vi "FGV PMA Kalibrieren.vi"(8 "GT?":bool, 10 "Aktionen PMA kalibrieren":T1, 11 "Sprachliste":string[][](array[string])) -> (1 "Zustand PMA":string, 2 "Aktionen PMA kalibrieren":T1)   [LabVIEW 2020, in "Auto Kalibrieren.lvlib"]
uses:
  Auto Kalibrieren.lvlib
  Aktionen PMA kalibrieren.ctl
  Aktion FGV CalZustand.ctl
  Analysator Definition/FGV Analysator Definition Aktionen.ctl
  Seiten/CalGas Aufschaltung/FGV CalGas Aktionen.ctl
  Seiten/EL3000/PMA/Aktion FGV Messwerte.ctl
  Aktionen FGV Zustand Kalibrierung.ctl
  Aktionen FGV AutoKAL Daten.ctl
  Seiten/EL3000/Allgemeine VI/FGV Uras26 Aktion.ctl
  Seiten/EL3000/PMA/Kalibrieren/Kalibrierung O2.ctl
  Seiten/EL3000/PMA/PMA.lvlib
  Seiten/EL3000/PMA/Kalibrieren/Kalibrieren.lvlib
  Seiten/EL3000/Allgemeine VI/Allgemeine VI.lvlib
  Analysator Definition/Analysator Definition.lvlib
  Seiten/CalGas Aufschaltung/CalGas Aufschaltung.lvlib
  Linearisierung V2/Linearisierung v2.lvlib
  Sprachverwaltung/Sprachverwaltung.lvlib
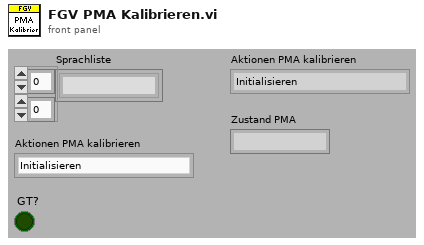
[diagram p1: front panel]
types:
  T1 = typedef "Auto Kalibrieren.lvlib/Aktionen PMA kalibrieren.ctl" = enum16{"Initialisieren", "Warten auf FT-IR", "Anstehende Störung", "0-Gas Aufschalten", "Nullpunkt Anfordern", "Nullpunkt", "Warten auf andere Messgeräte", "Messgas Aufschalten", "Endpunkt Anfordern", "Endpunkt", "Fertig", "Speichern"}
  T2 = typedef "Auto Kalibrieren.lvlib/Aktion FGV CalZustand.ctl" = enum16{"lesen", "Cal FTIR", "Cal FID CH4", "Cal PMA", "init", "Cal FID THC", "THC CG Eingang"}
  T3 = typedef "Analysator Definition.lvlib/FGV Analysator Definition Aktionen.ctl" = enum16{"lesen", "MB setzen", "MB KAL setzen", "laden"}
  T4 = typedef "CalGas Aufschaltung.lvlib/FGV CalGas Aktionen.ctl" = enum16{"lesen", "Analysator Auswahl", "Def.CalGas", "Aufschaltung CalGas", "laden", "speichern", "KAL extrahieren"}
  T5 = typedef "ABB-EL3000.lvlib/PMA.lvlib/Aktion FGV Messwerte.ctl" = enum16{"lesen", "Messwerte", "Messbereich", "Status", "Diagnose Werte"}
  T6 = typedef "Auto Kalibrieren.lvlib/Aktionen FGV Zustand Kalibrierung.ctl" = enum16{"lesen", "LÖSCHEN", "Hintergrund fertig", "Nullpunkt NDIR CO lo", "Endpunkt NDIR CO lo", "Nullpunkt NDIR CO hi", "Endpunkt NDIR CO hi", "Nullpunkt NDIR CO2 lo", "Endpunkt NDIR CO2 lo", "Nullpunkt FID CH4", "Endpunkt FID CH4", "Nullpunkt FID THC", "Endpunkt FID THC", "Nullpunkt PMA", "Endpunkt PMA", "Fehler FT-IR", "Fehler NDIR lo", "Fehler FID CH4", "Fehler FID THC", "Fehler PMA", "TIMEOUT"}
  T7 = typedef "Auto Kalibrieren.lvlib/Aktionen FGV AutoKAL Daten.ctl" = enum16{"lesen", "laden", "speichern", "Aufschaltzeit"}
  T8 = typedef "ABB-EL3000.lvlib/PMA.lvlib/Kalibrieren.lvlib/Kalibrierung O2.ctl" = enum16{"Nullpunkt O2", "Endpunkt O2"}
  T9 = typedef "ABB-EL3000.lvlib/Allgemeine VI.lvlib/FGV Uras26 Aktion.ctl" = enum16{"lesen", "CAL-Daten laden", "Messen", "Kalibrieren vorbereiten", "Kalibrieren", "CAL-Daten speichern", "Toleranz schreiben", "CAL-Daten kopieren"}
  T10 = typedef "Analysator Definition.lvlib/Betriebsdaten Komponente.ctl" = cluster{"Namen":string[], "MB Namen":string[], "Einheit":string, "MB Aktuell":u16, "MB Endwert":u16, "CalGase":u16[], "MB für KAL":u16[], "CG für KAL":u16[]}
  T11 = typedef "CalGas Aufschaltung.lvlib/Aufschaltung CalGas.ctl" = cluster{"Kalibriergas":T12, "Aufschaltpunkt":T13, "Analysator":T14}
  T12 = typedef "Auswahlfeld.ctl" = u16
  T13 = typedef "CalGas Aufschaltung.lvlib/Auswahl Aufschaltpunkt.ctl" = enum16{"über Filterblock", "Analysator direkt", "über PNS", "Entnahme", "Gasdivider"}
  T14 = typedef "CalGas Aufschaltung.lvlib/Auswahl Analysator.ctl" = enum16{"FT-IR", "FID", "PMA", "PMA/FID/FT-IR"}
  T15 = cluster{"Ausfall":bool, "Funktionskontrolle":bool, "Wartungsbedarf":bool}
  T16 = typedef "Auto Kalibrieren.lvlib/Auschaltzeiten Null Endpunktgase.ctl" = cluster{"CO lo 0":sgl, "CO lo E":sgl, "CO hi 0":sgl, "CO hi E":sgl, "CO2 lo 0":sgl, "CO2 lo E":sgl, "CH4 0":sgl, "CH4 E":sgl, "THC 0":sgl, "THC E":sgl, "O2 0":sgl, "O2 E":sgl}
  T17 = typedef "Auto Kalibrieren.lvlib/Zustand Messgeraete Kalibrierung.ctl" = cluster{"Hintergrund FT-IR":bool, "Nullpunkt NDIR CO lo":bool, "Endpunkt NDIR CO lo":bool, "Nullpunkt NDIR CO hi":bool, "Endpunkt NDIR CO hi":bool, "Nullpunkt NDIR CO2 lo":bool, "Endpunkt NDIR CO2 lo":bool, "Nullpunkt FID CH4":bool, "Endpunkt FID CH4":bool, "Nullpunkt FID THC":bool, "Endpunkt FID THC":bool, "Nullpunkt PMA":bool, "Endpunkt PMA":bool, "Fehler FT-IR":bool, "Fehler NDIR lo":bool, "Fehler FID CH4":bool, "Fehler FID THC":bool, "Fehler PMA":bool}
  T18 = typedef "Zahlen-Ausgabefeld.ctl" = sgl
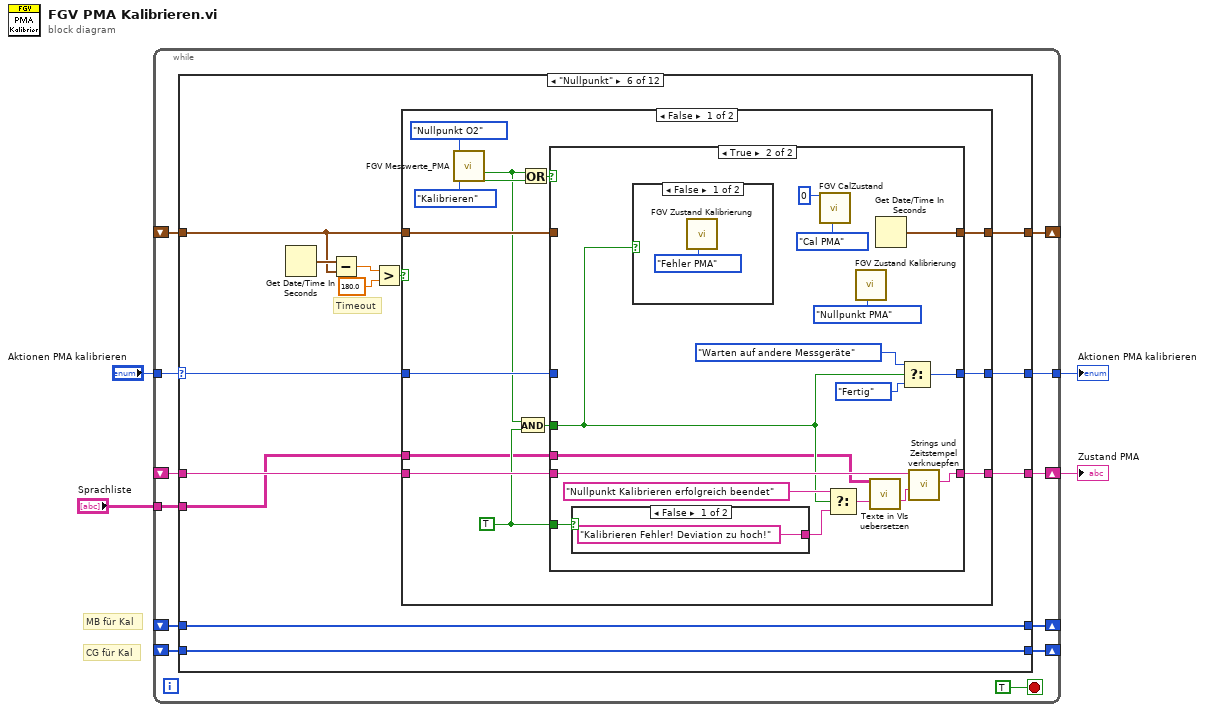
[diagram p0: block diagram]
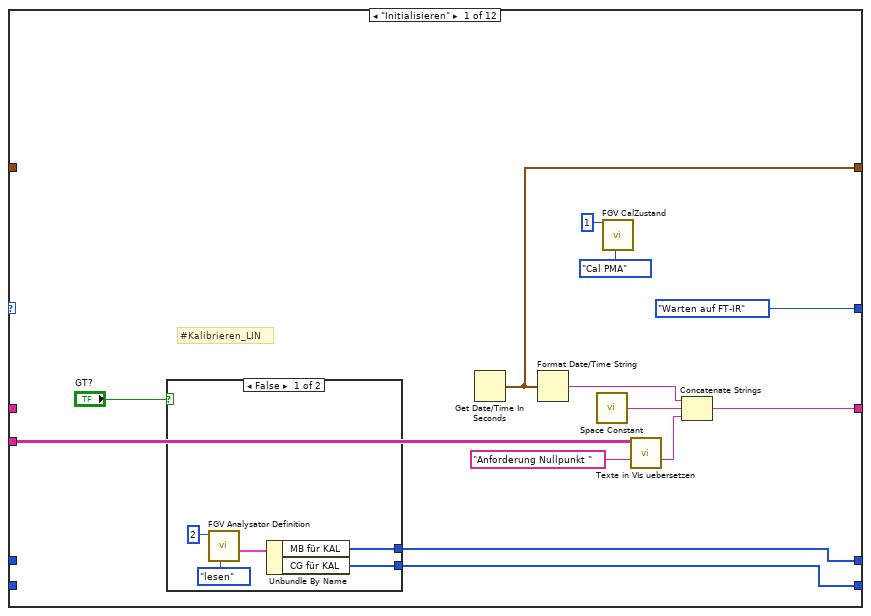
[diagram p2: hidden frame]
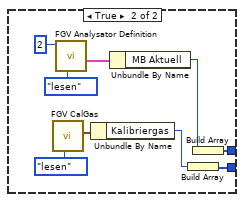
[diagram p3: hidden frame]
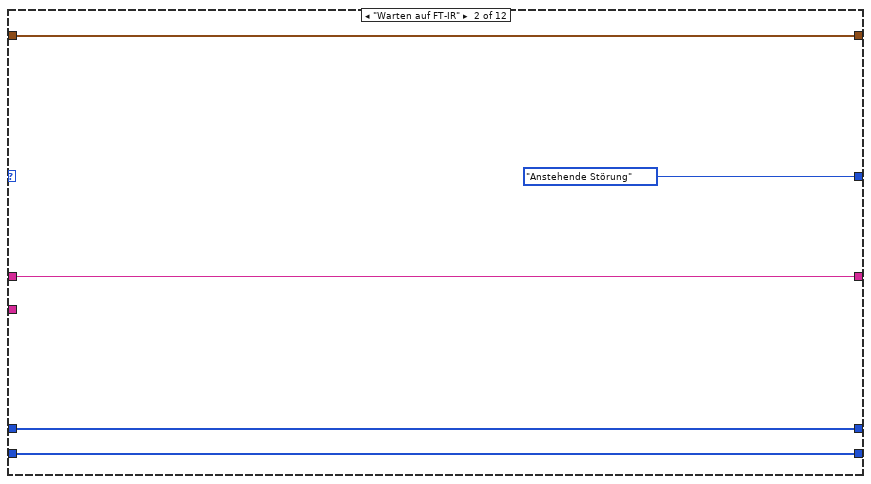
[diagram p4: hidden frame]
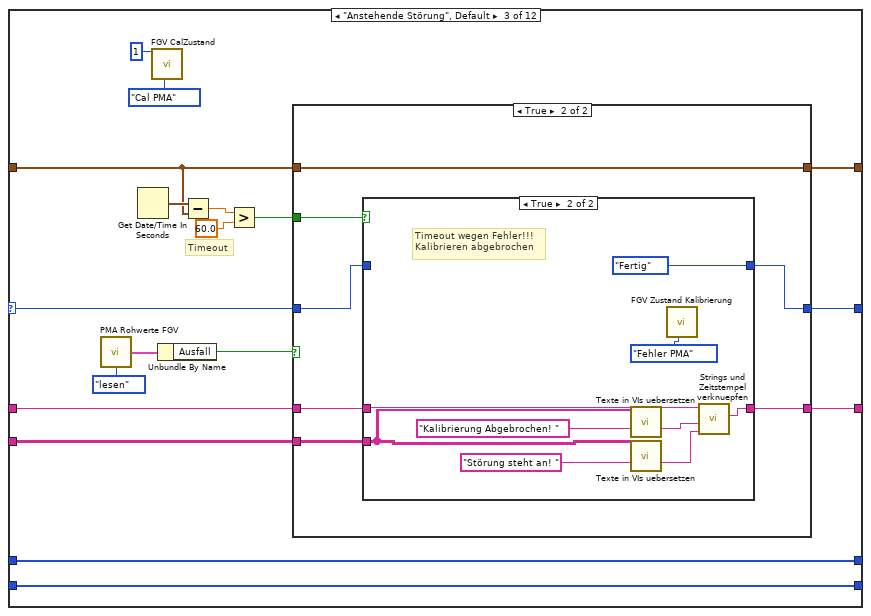
[diagram p5: hidden frame]
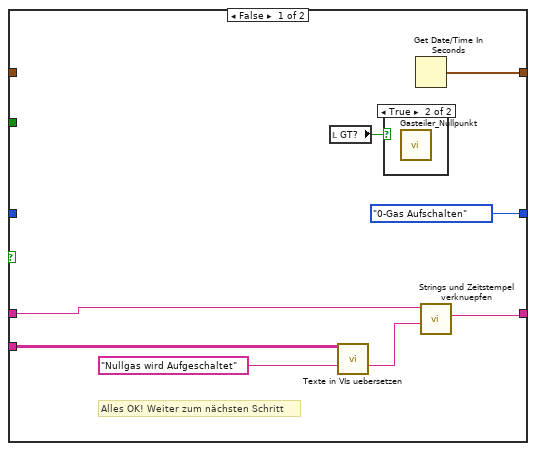
[diagram p6: hidden frame]
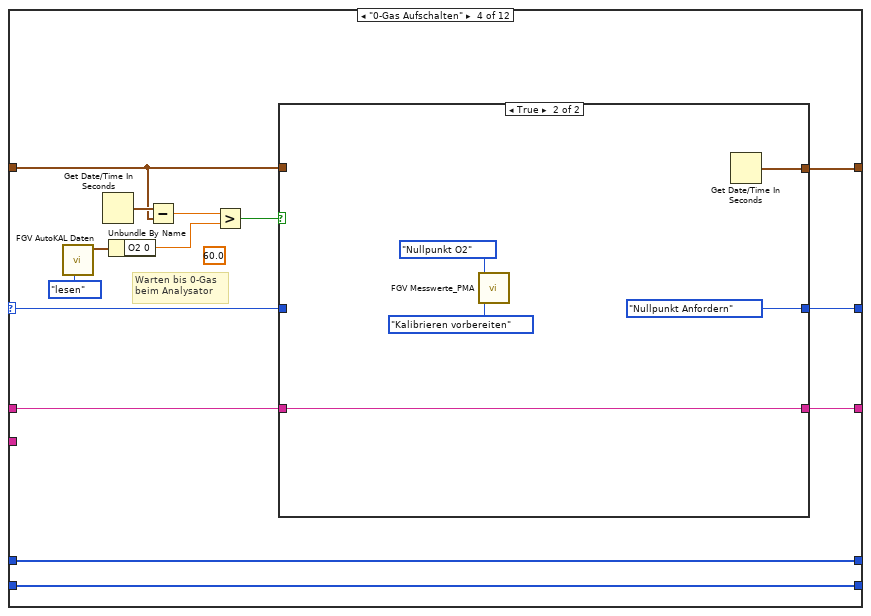
[diagram p9: hidden frame]
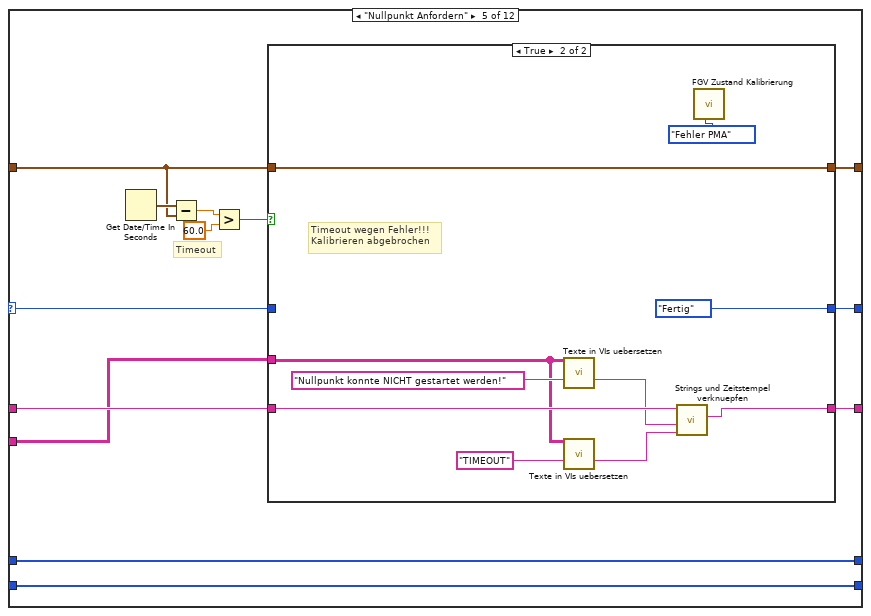
[diagram p11: hidden frame]
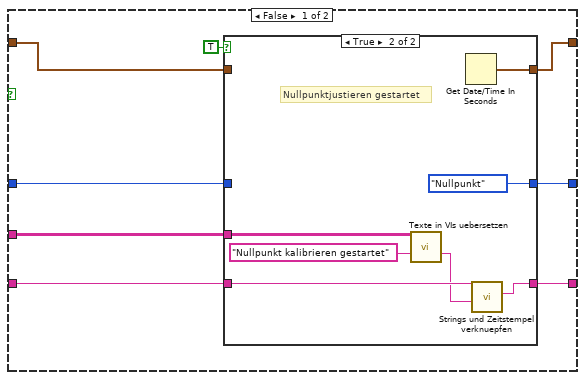
[diagram p12: hidden frame]
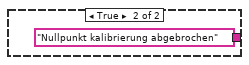
[diagram p15: hidden frame]
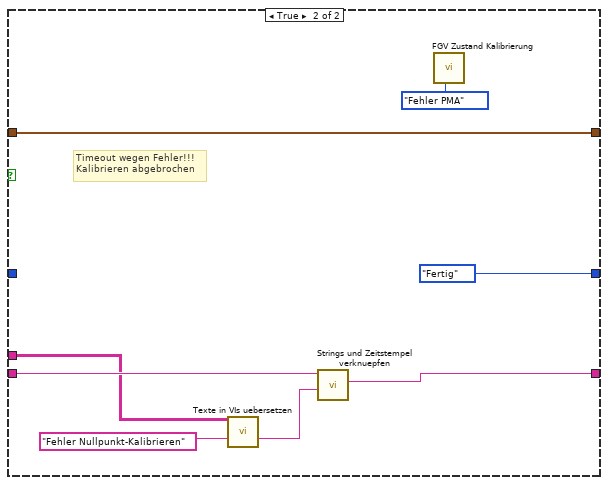
[diagram p17: hidden frame]
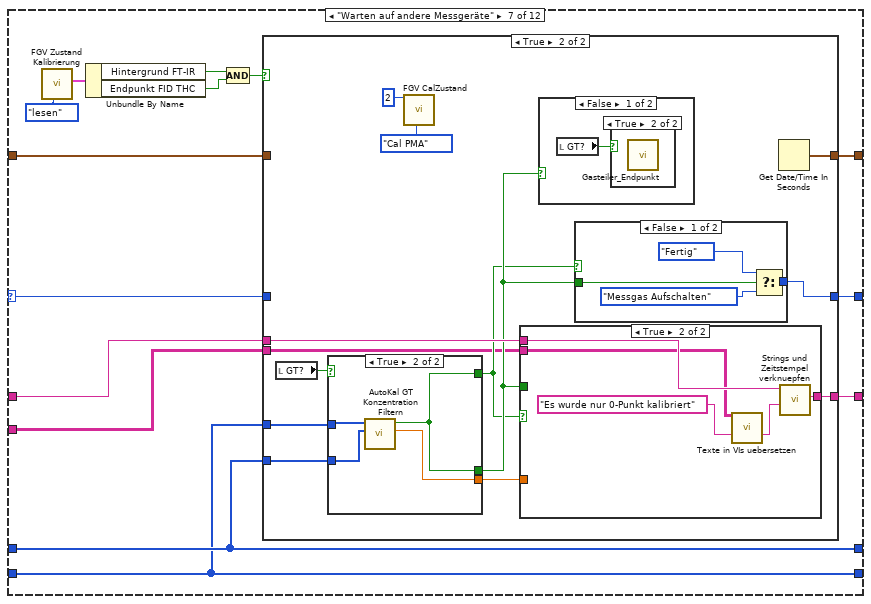
[diagram p18: hidden frame]
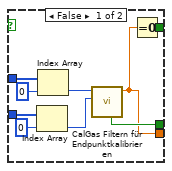
[diagram p20: hidden frame]
diagram:
  # "CG für Kal"
  # "MB für Kal"
  n1 = while {
    shift-right: [w12] -> w4
    shift-left: _ -> [w14]
    shift-right: [w13] -> _
    shift-left: _ -> [w15]
    tunnel: "Aktionen PMA kalibrieren" -> [w16]
    tunnel: [w11] -> w3
    shift-right: [w8] -> _
    shift-left: _ -> [w6]
    shift-right: [w9] -> _
    shift-left: _ -> [w7]
    tunnel: "Sprachliste" -> [w5]
    stop <- TRUE stop-if-true
    n2 = case shown="\"Nullpunkt\"" w16 {
      selector: w16 -> [_ _ w59 w101 w118 w159 w221 w295 w334 w379 w436 _]
      tunnel: w15 -> [_ w46 w57 w103 w123 w161 w222 w298 w339 w381 w437 _]
      tunnel: w14 -> [_ w48 w62 w99 w120 w163 w224 w293 w336 w380 w435 w444]
      tunnel: [w27 w46 w63 w102 w122 w160 w225 w297 w338 w378 w437 w446] -> w13
      tunnel: [w26 w48 w61 w98 w119 w162 w223 w292 w335 w376 w435 w444] -> w12
      tunnel: [Aktionen_PMA_kalibrieren."Warten auf FT-IR" ("Aktionen PMA kalibrieren") Aktionen_PMA_kalibrieren."Anstehende Störung" ("Aktionen PMA kalibrieren") w58 w100 w121 w164 w226 w294 w337 w377 w436 Aktionen_PMA_kalibrieren."Fertig" ("Aktionen PMA kalibrieren")] -> w11
      tunnel: [w24 w45 w52 w94 w117 w158 w217 w287 w333 w374 w429 w441] -> w9
      tunnel: [w23 w44 w51 w93 w116 w157 w216 w288 w332 w373 w428 w440] -> w8
      tunnel: w7 -> [_ w45 w52 w94 w117 w158 w217 w287 w333 w374 w429 w441]
      tunnel: w6 -> [_ w44 w51 w93 w116 w157 w216 w288 w332 w373 w428 w440]
      tunnel: w5 -> [w17 _ w49 _ w115 w156 w213 w286 w331 w372 _ _]
      frame "Initialisieren" {
        # "#Kalibrieren_LIN"
        n3 = case shown="False" "GT?" {
          tunnel: [w34 w35] -> w24
          tunnel: [w33 w40] -> w23
          frame False {
            n4 = call "FGV Analysator Definition.vi"("Aktionen"=FGV_Analysator_Definition_Aktionen."lesen", "Komponente"=2) -> ("Betriebsdaten Komponente"=w31:T10)  [unwired: 5 in, 4 out]
            n5 = Unbundle By Name(w31) -> ("MB für KAL"=w34:u16[], "CG für KAL"=w33:u16[])
          }
          frame True {
            n6 = call "FGV CalGas.vi"("Aktionen"=FGV_CalGas_Aktionen."lesen") -> ("Aufschaltung CalGas"=w42:T11)  [unwired: 6 in, 4 out]
            n7 = call "FGV Analysator Definition.vi"("Aktionen"=FGV_Analysator_Definition_Aktionen."lesen", "Komponente"=2) -> ("Betriebsdaten Komponente"=w39:T10)  [unwired: 5 in, 4 out]
            n8 = Unbundle By Name(w42) -> ("Kalibriergas"=w41:T12)
            n9 = Unbundle By Name(w39) -> ("MB Aktuell"=w36:u16)
            n10 = Build Array(w41) -> (w40:T12[])
            n11 = Build Array(w36) -> (w35:u16[])
          }
        }
        n12 = Get Date/Time In Seconds() -> (seconds since 1Jan1904=w27:timestamp)
        n13 = Format Date/Time String(seconds (now)=w27) -> (date/time string=w29:string)  [unwired: 2 in]
        n14 = call <vilib>:"Space Constant.vi"() -> ("String"=w28:string)
        n15 = call "FGV CalZustand.vi"("CAL Zustand"=u16 1 ("CAL Zustand FTIR"), "Aktion"=Aktion_FGV_CalZustand."Cal PMA") -> ()  [unwired: 13 in, 5 out]
        n16 = call "Texte in VIs uebersetzen.vi"("Sprachliste"=w17, "String zum Übersetzen"="Anforderung Nullpunkt " ("String")) -> ("String zum Übersetzen"=w18:string)  [unwired: 9 in, 4 out]
        n17 = Concatenate Strings(w29, w28, w18) -> (w26:string)
      }
      frame "Warten auf FT-IR" {
      }
      frame "Anstehende Störung", Default {
        # "Timeout"
        n18 = call "PMA Rohwerte FGV.vi"("Aktion"=Aktion_FGV_Messwerte."lesen") -> ("Status"=w55:T15)  [unwired: 11 in, 3 out]
        n19 = Get Date/Time In Seconds() -> (seconds since 1Jan1904=w66:timestamp)
        n20 = call "FGV CalZustand.vi"("CAL Zustand"=u16 1 ("CAL Zustand FTIR"), "Aktion"=Aktion_FGV_CalZustand."Cal PMA") -> ()  [unwired: 13 in, 5 out]
        n21 = Unbundle By Name(w55) -> ("Ausfall"=w56:bool)
        n22 = Subtract(x=w66, y=w57) -> (x-y=w65:dbl)
        n23 = Greater?(x=w65, y=60.0) -> (0:w60:bool)
        n24 = case shown="True" w56 {
          tunnel: [w74 w78] -> w63
          tunnel: w62 -> [w73 w77]
          tunnel: [w72 w76] -> w61
          tunnel: w60 -> [_ w81]
          tunnel: w59 -> [_ w80]
          tunnel: [Aktionen_PMA_kalibrieren."0-Gas Aufschalten" ("Aktionen PMA kalibrieren") w79] -> w58
          tunnel: w57 -> [_ w78]
          tunnel: w49 -> [w67 w75]
          frame False {
            # "Alles OK! Weiter zum nächsten Schritt"
            n25 = local read "GT?"() -> (w70:bool)
            n26 = call "Texte in VIs uebersetzen.vi"("Sprachliste"=w67, "String zum Übersetzen"="Nullgas wird Aufgeschaltet" ("String 1 hinzufügen")) -> ("String zum Übersetzen"=w68:string)  [unwired: 9 in, 4 out]
            n27 = case shown="True" w70 {
              frame False {
              }
              frame True {
                n28 = call "Gasteiler_Nullpunkt.vi"() -> ()  [unwired: 12 in]
              }
            }
            n29 = Get Date/Time In Seconds() -> (seconds since 1Jan1904=w74:timestamp)
            n30 = call "Strings und Zeitstempel verknuepfen.vi"("String 1 hinzufügen"=w68, "Eingagns String"=w73) -> ("Verknüpfter String"=w72:string)  [unwired: 9 in]
          }
          frame True {
            n31 = case shown="True" w81 {
              tunnel: w80 -> [w83 _]
              tunnel: [w83 Aktionen_PMA_kalibrieren."Fertig" ("Aktionen PMA kalibrieren")] -> w79
              tunnel: w77 -> [w82 w91]
              tunnel: [w82 w90] -> w76
              tunnel: w75 -> [_ w84]
              frame False {
                # "Fehler steht an!!!!"
              }
              frame True {
                # "Timeout wegen Fehler!!! \nKalibrieren abgebrochen"
                n32 = call "Texte in VIs uebersetzen.vi"("Sprachliste"=w84, "String zum Übersetzen"="Kalibrierung Abgebrochen! " ("String")) -> ("String zum Übersetzen"=w87:string)  [unwired: 9 in, 4 out]
                n33 = call "Texte in VIs uebersetzen.vi"("Sprachliste"=w84, "String zum Übersetzen"="Störung steht an! " ("String")) -> ("String zum Übersetzen"=w85:string)  [unwired: 9 in, 4 out]
                n34 = call "FGV Zustand Kalibrierung.vi"("Aktionen"=Aktionen_FGV_Zustand_Kalibrierung."Fehler PMA" ("Enum")) -> ()  [unwired: 9 in, 2 out]
                n35 = call "Strings und Zeitstempel verknuepfen.vi"("String 2 hinzufügen"=w85, "String 1 hinzufügen"=w87, "Eingagns String"=w91) -> ("Verknüpfter String"=w90:string)  [unwired: 8 in]
              }
            }
          }
        }
      }
      frame "0-Gas Aufschalten" {
        (unwired) 60.0 ("y")
        # "Warten bis 0-Gas \nbeim Analysator"
        n36 = call "FGV AutoKAL Daten.vi"("Aktionen"=Aktionen_FGV_AutoKAL_Daten."lesen") -> ("Aufschaltzeiten"=w96:T16)  [unwired: 10 in]
        n37 = Get Date/Time In Seconds() -> (seconds since 1Jan1904=w106:timestamp)
        n38 = Unbundle By Name(w96) -> ("O2 0"=w95:sgl)
        n39 = Subtract(x=w106, y=w103) -> (x-y=w105:dbl)
        n40 = Greater?(x=w105, y=w95) -> (0:w104:bool)
        n41 = case shown="True" w104 {
          tunnel: w103 -> [w109 _]
          tunnel: [w109 w114] -> w102
          tunnel: w101 -> [w108 _]
          tunnel: [w108 Aktionen_PMA_kalibrieren."Nullpunkt Anfordern" ("Aktionen PMA kalibrieren")] -> w100
          tunnel: w99 -> [w107 w113]
          tunnel: [w107 w113] -> w98
          frame False {
          }
          frame True {
            n42 = call "FGV Messwerte_PMA.vi"("Kalibrieren"=Kalibrierung_O2."Nullpunkt O2", "Aktion"=FGV_Uras26_Aktion."Kalibrieren vorbereiten") -> ()  [unwired: 18 in, 8 out]
            n43 = Get Date/Time In Seconds() -> (seconds since 1Jan1904=w114:timestamp)
          }
        }
      }
      frame "Nullpunkt Anfordern" {
        # "Timeout"
        n44 = Get Date/Time In Seconds() -> (seconds since 1Jan1904=w127:timestamp)
        n45 = Subtract(x=w127, y=w123) -> (x-y=w126:dbl)
        n46 = Greater?(x=w126, y=60.0) -> (0:w124:bool)
        n47 = case shown="True" w124 {
          tunnel: w123 -> [w131 w155]
          tunnel: [w130 w155] -> w122
          tunnel: [w133 Aktionen_PMA_kalibrieren."Fertig" ("Aktionen PMA kalibrieren")] -> w121
          tunnel: w120 -> [w135 w153]
          tunnel: [w134 w152] -> w119
          tunnel: w118 -> [w132 _]
          tunnel: w115 -> [w128 w146]
          frame False {
            n48 = case shown="True" TRUE {
              tunnel: w135 -> [w136 w145]
              tunnel: [w136 w144] -> w134
              tunnel: [w138 Aktionen_PMA_kalibrieren."Nullpunkt" ("Aktionen PMA kalibrieren")] -> w133
              tunnel: w132 -> [w138 _]
              tunnel: w131 -> [w137 _]
              tunnel: [w137 w142] -> w130
              tunnel: w128 -> [_ w139]
              frame False {
              }
              frame True {
                # "Nullpunktjustieren gestartet"
                n49 = call "Texte in VIs uebersetzen.vi"("Sprachliste"=w139, "String zum Übersetzen"="Nullpunkt kalibrieren gestartet" ("String 1 hinzufügen")) -> ("String zum Übersetzen"=w140:string)  [unwired: 9 in, 4 out]
                n50 = Get Date/Time In Seconds() -> (seconds since 1Jan1904=w142:timestamp)
                n51 = call "Strings und Zeitstempel verknuepfen.vi"("String 1 hinzufügen"=w140, "Eingagns String"=w145) -> ("Verknüpfter String"=w144:string)  [unwired: 9 in]
              }
            }
          }
          frame True {
            # "Timeout wegen Fehler!!! \nKalibrieren abgebrochen"
            n52 = call "Texte in VIs uebersetzen.vi"("Sprachliste"=w146, "String zum Übersetzen"="Nullpunkt konnte NICHT gestartet werden!" ("String")) -> ("String zum Übersetzen"=w149:string)  [unwired: 9 in, 4 out]
            n53 = call "Texte in VIs uebersetzen.vi"("Sprachliste"=w146, "String zum Übersetzen"="TIMEOUT" ("String")) -> ("String zum Übersetzen"=w147:string)  [unwired: 9 in, 4 out]
            n54 = call "Strings und Zeitstempel verknuepfen.vi"("String 2 hinzufügen"=w147, "String 1 hinzufügen"=w149, "Eingagns String"=w153) -> ("Verknüpfter String"=w152:string)  [unwired: 8 in]
            n55 = call "FGV Zustand Kalibrierung.vi"("Aktionen"=Aktionen_FGV_Zustand_Kalibrierung."Fehler PMA" ("Enum")) -> ()  [unwired: 9 in, 2 out]
          }
        }
      }
      frame "Nullpunkt" {
        # "Timeout"
        n56 = Get Date/Time In Seconds() -> (seconds since 1Jan1904=w168:timestamp)
        n57 = Subtract(x=w168, y=w161) -> (x-y=w167:dbl)
        n58 = Greater?(x=w167, y=180.0) -> (0:w165:bool)
        n59 = case shown="False" w165 {
          tunnel: [w179 Aktionen_PMA_kalibrieren."Fertig" ("Aktionen PMA kalibrieren")] -> w164
          tunnel: w163 -> [w178 w211]
          tunnel: [w177 w210] -> w162
          tunnel: w161 -> [w182 w209]
          tunnel: [w181 w209] -> w160
          tunnel: w159 -> [w180 _]
          tunnel: w156 -> [w169 w205]
          frame False {
            w172 = TRUE
            n60 = call "FGV Messwerte_PMA.vi"("Kalibrieren"=Kalibrierung_O2."Nullpunkt O2", "Aktion"=FGV_Uras26_Aktion."Kalibrieren") -> ("Kalibrieren erfolgreich"=w174:bool, "CAL TimeOut"=w175:bool)  [unwired: 18 in, 6 out]
            n61 = And(x=w174, y=w172) -> (x .and. y?=w173:bool)
            n62 = Or(x=w174, y=w175) -> (x .or. y?=w176:bool)
            n63 = case shown="True" w176 {
              tunnel: w182 -> [w185 _]
              tunnel: [w185 w194] -> w181
              tunnel: w180 -> [w184 _]
              tunnel: [w184 w195] -> w179
              tunnel: w178 -> [w183 w201]
              tunnel: [w183 w200] -> w177
              tunnel: w173 -> [_ w192]
              tunnel: w172 -> [_ w191]
              tunnel: w169 -> [_ w186]
              frame False {
              }
              frame True {
                n64 = case shown="False" w191 {
                  tunnel: ["Kalibrieren Fehler! Deviation zu hoch!" ("String 1 hinzufügen") "Nullpunkt kalibrierung abgebrochen" ("String 1 hinzufügen")] -> w198
                  frame False {
                  }
                  frame True {
                  }
                }
                n65 = case shown="False" w192 {
                  frame False {
                    n66 = call "FGV Zustand Kalibrierung.vi"("Aktionen"=Aktionen_FGV_Zustand_Kalibrierung."Fehler PMA" ("Enum")) -> ()  [unwired: 9 in, 2 out]
                  }
                  frame True {
                  }
                }
                n67 = call "FGV CalZustand.vi"("CAL Zustand"=u16 0 ("CAL Zustand FTIR"), "Aktion"=Aktion_FGV_CalZustand."Cal PMA") -> ()  [unwired: 13 in, 5 out]
                n68 = Select(t="Nullpunkt Kalibrieren erfolgreich beendet" ("String 1 hinzufügen"), s=w192, f=w198) -> (s? t:f=w188:string)
                n69 = call "FGV Zustand Kalibrierung.vi"("Aktionen"=Aktionen_FGV_Zustand_Kalibrierung."Nullpunkt PMA" ("Enum")) -> ()  [unwired: 9 in, 2 out]
                n70 = call "Texte in VIs uebersetzen.vi"("Sprachliste"=w186, "String zum Übersetzen"=w188) -> ("String zum Übersetzen"=w187:string)  [unwired: 9 in, 4 out]
                n71 = Get Date/Time In Seconds() -> (seconds since 1Jan1904=w194:timestamp)
                n72 = Select(t=Aktionen_PMA_kalibrieren."Warten auf andere Messgeräte" ("Aktionen PMA kalibrieren"), s=w192, f=Aktionen_PMA_kalibrieren."Fertig" ("Aktionen PMA kalibrieren")) -> (s? t:f=w195:T1)
                n73 = call "Strings und Zeitstempel verknuepfen.vi"("String 1 hinzufügen"=w187, "Eingagns String"=w201) -> ("Verknüpfter String"=w200:string)  [unwired: 9 in]
              }
            }
          }
          frame True {
            # "Timeout wegen Fehler!!! \nKalibrieren abgebrochen"
            n74 = call "Texte in VIs uebersetzen.vi"("Sprachliste"=w205, "String zum Übersetzen"="Fehler Nullpunkt-Kalibrieren" ("String 1 hinzufügen")) -> ("String zum Übersetzen"=w206:string)  [unwired: 9 in, 4 out]
            n75 = call "Strings und Zeitstempel verknuepfen.vi"("String 1 hinzufügen"=w206, "Eingagns String"=w211) -> ("Verknüpfter String"=w210:string)  [unwired: 9 in]
            n76 = call "FGV Zustand Kalibrierung.vi"("Aktionen"=Aktionen_FGV_Zustand_Kalibrierung."Fehler PMA" ("Enum")) -> ()  [unwired: 9 in, 2 out]
          }
        }
      }
      frame "Warten auf andere Messgeräte" {
        n77 = call "FGV Zustand Kalibrierung.vi"("Aktionen"=Aktionen_FGV_Zustand_Kalibrierung."lesen" ("Enum")) -> ("Zustand Kalibrierung"=w219:T17)  [unwired: 9 in, 1 out]
        n78 = Unbundle By Name(w219) -> ("Hintergrund FT-IR"=w218:bool, "Endpunkt FID THC"=w214:bool)
        n79 = Compound Arithmetic op=AND(w218, w214) -> (w215:bool)
        n80 = case shown="True" w215 {
          tunnel: [w228 w239] -> w226
          tunnel: [w229 w242] -> w225
          tunnel: w224 -> [w227 w241]
          tunnel: [w227 w240] -> w223
          tunnel: w222 -> [w229 _]
          tunnel: w221 -> [w228 _]
          tunnel: w216 -> [_ w236]
          tunnel: w217 -> [_ w235]
          tunnel: w213 -> [_ w230]
          frame False {
          }
          frame True {
            n81 = local read "GT?"() -> (w231:bool)
            n82 = case shown="True" w231 {
              tunnel: w236 -> [w251 w253]
              tunnel: w235 -> [w249 w252]
              tunnel: [w245 w255] -> w234
              tunnel: [w244 w254] -> w233
              tunnel: [w243 w255] -> w232
              frame False {
                n83 = Index Array(array=w249, index=0 ("Index")) -> (element=w246:u16)
                n84 = Index Array(array=w251, index=0 ("Index")) -> (element=w247:T12)
                n85 = call "CalGas Filtern für Endpunktkalibrieren.vi"("Messbereich"=w246, "CalGas"=w247) -> ("Wert 1"=w244:T18, "Fehler"=w245:bool)  [unwired: 2 in, 6 out]
                n86 = Equal To 0?(x=w244) -> (x = 0?=w243:bool)
              }
              frame True {
                n87 = call "AutoKal GT Konzentration Filtern.vi"("CG für KAL"=w252, "MB für KAL"=w253) -> ("Konzentration"=w254:dbl, "Fehler/Leer"=w255:bool)  [unwired: 6 in, 2 out]
              }
            }
            n88 = call "FGV CalZustand.vi"("CAL Zustand"=u16 2 ("CAL Zustand FTIR"), "Aktion"=Aktion_FGV_CalZustand."Cal PMA") -> ()  [unwired: 13 in, 5 out]
            n89 = case shown="True" w232 {
              tunnel: w241 -> [w271 w278]
              tunnel: [w270 w277] -> w240
              tunnel: w234 -> [w265 _]
              tunnel: w233 -> [w264 _]
              tunnel: w230 -> [w257 w274]
              frame False {
                n90 = Number To Fractional String(number=w264, precision (6)=i16 3 ("Genauigkeit (6)")) -> (F-format string=w268:string)  [unwired: 2 in]
                n91 = call "Texte in VIs uebersetzen.vi"("Sprachliste"=w257, "String zum Übersetzen"="Endpunkt" ("String 1 hinzufügen")) -> ("Sprachliste out"=w256:string[][], "String zum Übersetzen"=w262:string)  [unwired: 9 in, 3 out]
                n92 = call "Texte in VIs uebersetzen.vi"("Sprachliste"=w257, "String zum Übersetzen"="Kein Prüfgas für O2 vorhanden" ("String 1 hinzufügen")) -> ("String zum Übersetzen"=w258:string)  [unwired: 9 in, 4 out]
                n93 = call "Texte in VIs uebersetzen.vi"("Sprachliste"=w256, "String zum Übersetzen"="(Konzentration: " ("String")) -> ("String zum Übersetzen"=w260:string)  [unwired: 9 in, 4 out]
                n94 = Concatenate Strings(w260, w268, ")" ("String")) -> (w272:string)
                n95 = call "Strings und Zeitstempel verknuepfen.vi"("String 2 hinzufügen"=w272, "String 1 hinzufügen"=w262, "Eingagns String"=w271) -> ("Verknüpfter String"=w266:string)  [unwired: 8 in]
                n96 = call "Strings und Zeitstempel verknuepfen.vi"("String 1 hinzufügen"=w258, "Eingagns String"=w271) -> ("Verknüpfter String"=w267:string)  [unwired: 9 in]
                n97 = Select(t=w267, s=w265, f=w266) -> (s? t:f=w270:string)
              }
              frame True {
                n98 = call "Texte in VIs uebersetzen.vi"("Sprachliste"=w274, "String zum Übersetzen"="Es wurde nur 0-Punkt kalibriert" ("String 1 hinzufügen")) -> ("String zum Übersetzen"=w275:string)  [unwired: 9 in, 4 out]
                n99 = call "Strings und Zeitstempel verknuepfen.vi"("String 1 hinzufügen"=w275, "Eingagns String"=w278) -> ("Verknüpfter String"=w277:string)  [unwired: 9 in]
              }
            }
            n100 = case shown="False" w234 {
              frame False {
                n101 = local read "GT?"() -> (w284:bool)
                n102 = case shown="True" w284 {
                  frame False {
                  }
                  frame True {
                    n103 = call "Gasteiler_Endpunkt.vi"() -> ()  [unwired: 12 in]
                  }
                }
              }
              frame True {
                n104 = call "FGV Zustand Kalibrierung.vi"("Aktionen"=Aktionen_FGV_Zustand_Kalibrierung."Fehler PMA" ("Enum")) -> ()  [unwired: 9 in, 2 out]
              }
            }
            n105 = case shown="False" w232 {
              tunnel: [w282 Aktionen_PMA_kalibrieren."Speichern" ("Aktionen PMA kalibrieren")] -> w239
              tunnel: w234 -> [w279 _]
              frame False {
                n106 = Select(t=Aktionen_PMA_kalibrieren."Fertig" ("f"), s=w279, f=Aktionen_PMA_kalibrieren."Messgas Aufschalten" ("Aktionen PMA kalibrieren")) -> (s? t:f=w282:T1)
              }
              frame True {
              }
            }
            n107 = Get Date/Time In Seconds() -> (seconds since 1Jan1904=w242:timestamp)
          }
        }
      }
      frame "Messgas Aufschalten" {
        n108 = call "FGV AutoKAL Daten.vi"("Aktionen"=Aktionen_FGV_AutoKAL_Daten."lesen") -> ("Aufschaltzeiten"=w290:T16)  [unwired: 10 in]
        n109 = Unbundle By Name(w290) -> ("O2 E"=w289:sgl)
        n110 = Get Date/Time In Seconds() -> (seconds since 1Jan1904=w300:timestamp)
        n111 = Subtract(x=w300, y=w298) -> (x-y=w299:dbl)
        n112 = Greater?(x=w299, y=w289) -> (0:w296:bool)
        n113 = case shown="False" w296 {
          tunnel: w298 -> [w303 _]
          tunnel: [w303 w317] -> w297
          tunnel: w295 -> [w302 _]
          tunnel: [w302 Aktionen_PMA_kalibrieren."Endpunkt Anfordern" ("Aktionen PMA kalibrieren")] -> w294
          tunnel: w293 -> [w301 w319]
          tunnel: [w301 w320] -> w292
          tunnel: w288 -> [_ w311]
          tunnel: w287 -> [_ w310]
          tunnel: w286 -> [_ w304]
          frame False {
          }
          frame True {
            n114 = local read "GT?"() -> (w309:bool)
            n115 = case shown="True" w309 {
              tunnel: [w325 w330] -> w312
              tunnel: w311 -> [w324 _]
              tunnel: w310 -> [w323 _]
              frame False {
                n116 = Index Array(array=w323, index=0 ("Index")) -> (element=w326:u16)
                n117 = Index Array(array=w324, index=0 ("Index")) -> (element=w327:T12)
                n118 = call "CalGas Filtern für Endpunktkalibrieren.vi"("Messbereich"=w326, "CalGas"=w327) -> ("Wert 1"=w325:T18)  [unwired: 2 in, 7 out]
              }
              frame True {
                n119 = call "AutoKal GT Konzentration Filtern.vi"() -> ("Konzentration"=w330:dbl)  [unwired: 8 in, 3 out]
              }
            }
            n120 = call "FGV Messwerte_PMA.vi"("Prüfgaskonz."=w312, "Kalibrieren"=Kalibrierung_O2."Endpunkt O2", "Aktion"=FGV_Uras26_Aktion."Kalibrieren vorbereiten") -> ()  [unwired: 17 in, 8 out]
            n121 = call "Texte in VIs uebersetzen.vi"("Sprachliste"=w304, "String zum Übersetzen"="(Konzentration: " ("String")) -> ("String zum Übersetzen"=w305:string)  [unwired: 9 in, 4 out]
            n122 = Number To Fractional String(number=w312, precision (6)=i16 3 ("Genauigkeit (6)")) -> (F-format string=w315:string)  [unwired: 2 in]
            n123 = call "Texte in VIs uebersetzen.vi"("Sprachliste"=w304, "String zum Übersetzen"="Anforderung Endpunkt kalibrieren" ("String 1 hinzufügen")) -> ("String zum Übersetzen"=w307:string)  [unwired: 9 in, 4 out]
            n124 = Concatenate Strings(w305, w315, ")" ("String")) -> (w321:string)
            n125 = Get Date/Time In Seconds() -> (seconds since 1Jan1904=w317:timestamp)
            n126 = call "Strings und Zeitstempel verknuepfen.vi"("String 2 hinzufügen"=w321, "String 1 hinzufügen"=w307, "Eingagns String"=w319) -> ("Verknüpfter String"=w320:string)  [unwired: 8 in]
          }
        }
      }
      frame "Endpunkt Anfordern" {
        # "Timeout"
        n127 = Get Date/Time In Seconds() -> (seconds since 1Jan1904=w343:timestamp)
        n128 = Subtract(x=w343, y=w339) -> (x-y=w342:dbl)
        n129 = Greater?(x=w342, y=100.0) -> (0:w340:bool)
        n130 = case shown="False" w340 {
          tunnel: w339 -> [w351 w371]
          tunnel: [w346 w371] -> w338
          tunnel: [w347 Aktionen_PMA_kalibrieren."Fertig" ("Aktionen PMA kalibrieren")] -> w337
          tunnel: w336 -> [w349 w369]
          tunnel: [w348 w368] -> w335
          tunnel: w334 -> [w350 _]
          tunnel: w331 -> [w344 w362]
          frame False {
            n131 = case shown="True" TRUE {
              tunnel: w349 -> [w352 w361]
              tunnel: [w352 w360] -> w348
              tunnel: [w354 Aktionen_PMA_kalibrieren."Endpunkt" ("Aktionen PMA kalibrieren")] -> w347
              tunnel: w350 -> [w354 _]
              tunnel: w351 -> [w353 _]
              tunnel: [w353 w358] -> w346
              tunnel: w344 -> [_ w355]
              frame False {
              }
              frame True {
                # "Endpunkt Kalibrieren gestartet"
                n132 = call "Texte in VIs uebersetzen.vi"("Sprachliste"=w355, "String zum Übersetzen"="Endpunkt kalibrieren gestartet" ("String 1 hinzufügen")) -> ("String zum Übersetzen"=w356:string)  [unwired: 9 in, 4 out]
                n133 = call "Strings und Zeitstempel verknuepfen.vi"("String 1 hinzufügen"=w356, "Eingagns String"=w361) -> ("Verknüpfter String"=w360:string)  [unwired: 9 in]
                n134 = Get Date/Time In Seconds() -> (seconds since 1Jan1904=w358:timestamp)
              }
            }
          }
          frame True {
            # "Timeout wegen Fehler!!! \nKalibrieren abgebrochen"
            n135 = call "FGV Zustand Kalibrierung.vi"("Aktionen"=Aktionen_FGV_Zustand_Kalibrierung."Fehler PMA" ("Enum")) -> ()  [unwired: 9 in, 2 out]
            n136 = call "Texte in VIs uebersetzen.vi"("Sprachliste"=w362, "String zum Übersetzen"="Endpunkt konnte NICHT gestartet werden!" ("String")) -> ("String zum Übersetzen"=w365:string)  [unwired: 9 in, 4 out]
            n137 = call "Texte in VIs uebersetzen.vi"("Sprachliste"=w362, "String zum Übersetzen"="TIMEOUT" ("String")) -> ("String zum Übersetzen"=w363:string)  [unwired: 9 in, 4 out]
            n138 = call "Strings und Zeitstempel verknuepfen.vi"("String 2 hinzufügen"=w363, "String 1 hinzufügen"=w365, "Eingagns String"=w369) -> ("Verknüpfter String"=w368:string)  [unwired: 8 in]
          }
        }
      }
      frame "Endpunkt" {
        # "Timeout"
        n139 = Get Date/Time In Seconds() -> (seconds since 1Jan1904=w384:timestamp)
        n140 = Subtract(x=w384, y=w381) -> (x-y=w383:dbl)
        n141 = Greater?(x=w383, y=180.0) -> (0:w375:bool)
        n142 = case shown="False" w375 {
          tunnel: [w395 Aktionen_PMA_kalibrieren."Fertig" ("Aktionen PMA kalibrieren")] -> w377
          tunnel: w380 -> [w394 w425]
          tunnel: [w393 w424] -> w376
          tunnel: w381 -> [w398 w423]
          tunnel: [w397 w423] -> w378
          tunnel: w379 -> [w396 _]
          tunnel: w372 -> [w385 w419]
          frame False {
            w388 = TRUE
            n143 = call "FGV Messwerte_PMA.vi"("Kalibrieren"=Kalibrierung_O2."Endpunkt O2", "Aktion"=FGV_Uras26_Aktion."Kalibrieren") -> ("Kalibrieren erfolgreich"=w390:bool, "CAL TimeOut"=w391:bool)  [unwired: 18 in, 6 out]
            n144 = Or(x=w390, y=w391) -> (x .or. y?=w392:bool)
            n145 = And(x=w390, y=w388) -> (x .and. y?=w389:bool)
            n146 = case shown="True" w392 {
              tunnel: w398 -> [w401 _]
              tunnel: [w401 w411] -> w397
              tunnel: w396 -> [w400 _]
              tunnel: [w400 w408] -> w395
              tunnel: w394 -> [w399 w415]
              tunnel: [w399 w414] -> w393
              tunnel: w389 -> [_ w406]
              tunnel: w388 -> [_ w405]
              tunnel: w385 -> [_ w402]
              frame False {
              }
              frame True {
                n147 = case shown="True" w405 {
                  tunnel: ["Kalibriern Fehler! Deviation zu Hoch!" ("String 1 hinzufügen") "Endpunkt Kalibrierung abgebrochen!" ("String 1 hinzufügen")] -> w412
                  frame False {
                  }
                  frame True {
                  }
                }
                n148 = case shown="False" w406 {
                  frame False {
                    n149 = call "FGV Zustand Kalibrierung.vi"("Aktionen"=Aktionen_FGV_Zustand_Kalibrierung."Fehler PMA" ("Enum")) -> ()  [unwired: 9 in, 2 out]
                  }
                  frame True {
                  }
                }
                n150 = Select(t="Endpunkt Kalibrierung erfolgreich beendet" ("String 1 hinzufügen"), s=w406, f=w412) -> (s? t:f=w404:string)
                n151 = Get Date/Time In Seconds() -> (seconds since 1Jan1904=w411:timestamp)
                n152 = call "FGV Zustand Kalibrierung.vi"("Aktionen"=Aktionen_FGV_Zustand_Kalibrierung."Endpunkt PMA" ("Enum")) -> ()  [unwired: 9 in, 2 out]
                n153 = call "Texte in VIs uebersetzen.vi"("Sprachliste"=w402, "String zum Übersetzen"=w404) -> ("String zum Übersetzen"=w403:string)  [unwired: 9 in, 4 out]
                n154 = Select(t=Aktionen_PMA_kalibrieren."Speichern", s=w406, f=Aktionen_PMA_kalibrieren."Fertig" ("Aktionen PMA kalibrieren")) -> (s? t:f=w408:T1)
                n155 = call "Strings und Zeitstempel verknuepfen.vi"("String 1 hinzufügen"=w403, "Eingagns String"=w415) -> ("Verknüpfter String"=w414:string)  [unwired: 9 in]
              }
            }
          }
          frame True {
            # "Timeout wegen Fehler!!! \nKalibrieren abgebrochen"
            n156 = call "FGV Zustand Kalibrierung.vi"("Aktionen"=Aktionen_FGV_Zustand_Kalibrierung."Fehler PMA" ("Enum")) -> ()  [unwired: 9 in, 2 out]
            n157 = call "Texte in VIs uebersetzen.vi"("Sprachliste"=w419, "String zum Übersetzen"="Fehler Endpunkt-Kalibrieren" ("String 1 hinzufügen")) -> ("String zum Übersetzen"=w420:string)  [unwired: 9 in, 4 out]
            n158 = call "Strings und Zeitstempel verknuepfen.vi"("String 1 hinzufügen"=w420, "Eingagns String"=w425) -> ("Verknüpfter String"=w424:string)  [unwired: 9 in]
          }
        }
      }
      frame "Fertig" {
        n159 = call "FGV Zustand Kalibrierung.vi"("Aktionen"=Aktionen_FGV_Zustand_Kalibrierung."lesen" ("Enum")) -> ("Zustand Kalibrierung"=w433:T17)  [unwired: 9 in, 1 out]
        n160 = Unbundle By Name(w433) -> ("Nullpunkt PMA"=w432:bool, "Endpunkt PMA"=w431:bool)
        n161 = And(x=w432, y=w431) -> (x .and. y?=w430:bool)
        n162 = case shown="True" w430 {
          frame False {
          }
          frame True {
            n163 = call "FGV CalZustand.vi"("CAL Zustand"=u16 0 ("CAL Zustand FTIR"), "Aktion"=Aktion_FGV_CalZustand."Cal PMA") -> ()  [unwired: 13 in, 5 out]
          }
        }
        n164 = local read "GT?"() -> (w427:bool)
        n165 = case shown="True" w427 {
          frame False {
          }
          frame True {
            n166 = call "Gasteiler_Standby.vi"() -> ()  [unwired: 12 in]
          }
        }
      }
      frame "Speichern" {
        n167 = call "FGV Zustand Kalibrierung.vi"("Aktionen"=Aktionen_FGV_Zustand_Kalibrierung."Endpunkt PMA" ("Enum")) -> ()  [unwired: 9 in, 2 out]
        n168 = call "FGV Messwerte_PMA.vi"("Aktion"=FGV_Uras26_Aktion."CAL-Daten speichern") -> ()  [unwired: 19 in, 8 out]
        n169 = Get Date/Time In Seconds() -> (seconds since 1Jan1904=w446:timestamp)
      }
    }
  }
  "Zustand PMA" <- w4
  "Aktionen PMA kalibrieren" <- w3
